vi "AlliGator Toggle Phasor Plot(s) Locking to Reference n.vi"(4 "Ref 1(F)/Ref 2(T)":bool, 6 "Phasor Frequency":dbl[unit], 7 "Phasor Graph Refnum":refnum<vi>, 8 "error in":errorcluster, 9 "State Indicators":refnum<vi>, 10 "Phasor Graph Ctrl Refnums":T1, 11 "[Phasor Plot(s) locked to Ref n] in":i32[](array[numeric])) -> (0 "error out":errorcluster, 3 "[Phasor Plot(s) locked to Ref n] out":i32[](array[numeric]))   [LabVIEW 2021, in "AlliGator Phasor Graph.lvlib"]
doc: "Locks Phasor Plot(s) to a reference."
uses:
  AlliGator Phasor Graph.lvlib
  AlliGator Phasor Graph Ctrl Refnums.ctl
  Phasor/Phasor Calibration Type.ctl
  AlliGator State Indicator.ctl
  AlliGator Variables List.ctl
  AlliGator Globals, Variables & Constants.lvlib
  Graphs/XY Graph/XY Graph Add-Ons.lvlib
  Sound/Sound.lvlib
  Phasor/Phasor.lvlib
  AlliGator GUI.lvlib
panel:
  # "see the AlliGator License on the block diagram (Ctrl+E or Window:Show Block Diagram)"
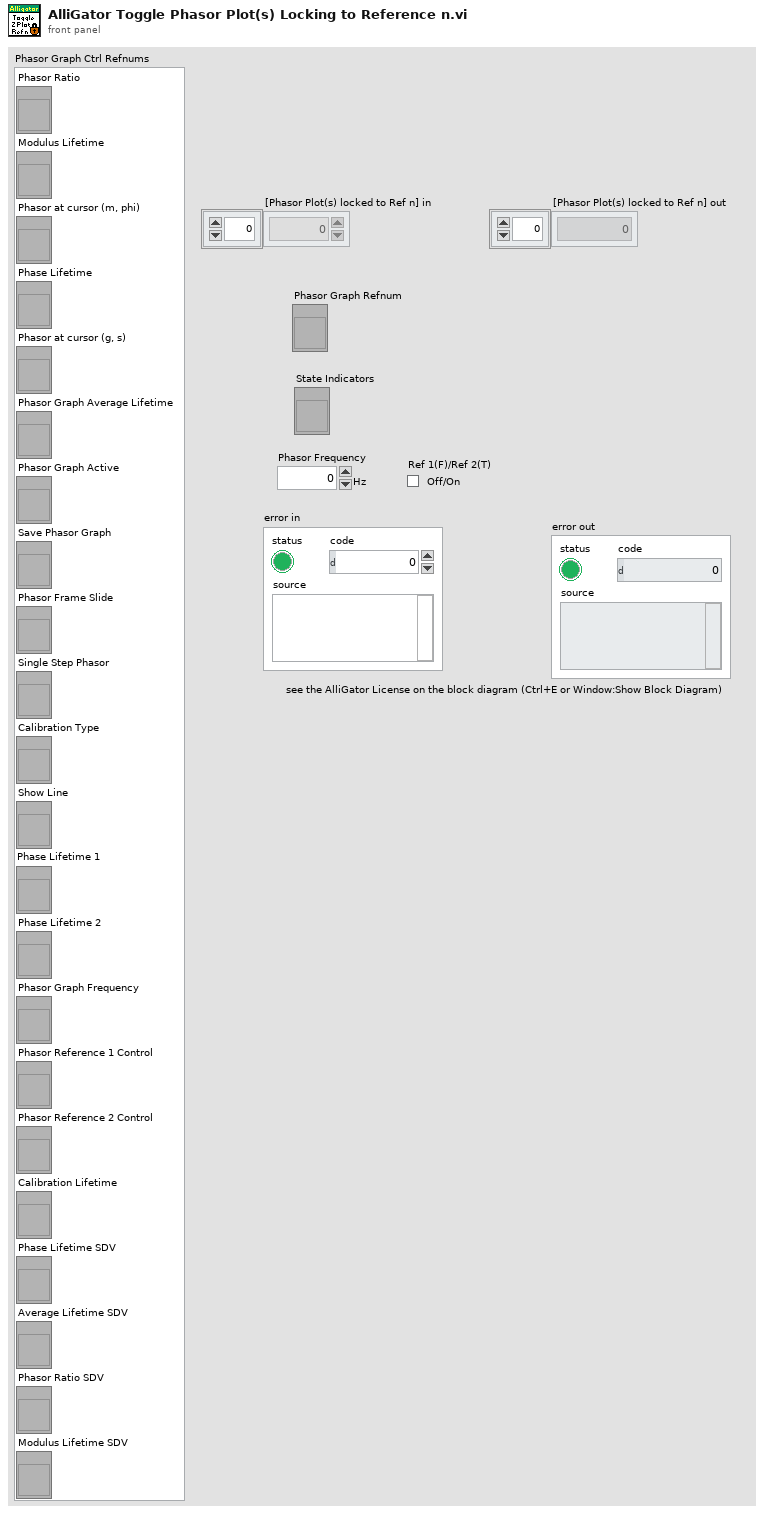
[diagram p1: front panel]
types:
  T1 = typedef "AlliGator GUI.lvlib/AlliGator Phasor Graph Ctrl Refnums.ctl" = cluster{"Phasor Ratio":refnum<vi>, "Modulus Lifetime":refnum<vi>, "Phasor at cursor (m, phi)":refnum<vi>, "Phase Lifetime":refnum<vi>, "Phasor at cursor (g, s)":refnum<vi>, "Phasor Graph Average Lifetime":refnum<vi>, "Phasor Graph Active":refnum<vi>, "Save Phasor Graph":refnum<vi>, "Phasor Frame Slide":refnum<vi>, "Single Step Phasor":refnum<vi>, "Calibration Type":refnum<vi>, "Show Line":refnum<vi>, "Phase Lifetime 1":refnum<vi>, "Phase Lifetime 2":refnum<vi>, "Phasor Graph Frequency":refnum<vi>, "Phasor Reference 1 Control":refnum<vi>, "Phasor Reference 2 Control":refnum<vi>, "Calibration Lifetime":refnum<vi>, "Phase Lifetime SDV":refnum<vi>, "Average Lifetime SDV":refnum<vi>, "Phasor Ratio SDV":refnum<vi>, "Modulus Lifetime SDV":refnum<vi>}
  T2 = typedef "AlliGator Globals, Variables & Constants.lvlib/AlliGator Variables List.ctl" = enum16{"---- GUI ----", "Initialization Status", "State Indicators Refnum", "Original AlliGator Menu Items", "Current Action Loop State", "Script in progress", "Playback", "Loop Playback", "Search ROI Used", "Search ROI", "Decay Graph Max Legend Size", "Intensity Graph Max Legend Size", "Decay Statistics Graph Max Legend Size", "Phasor Graph Max Legend Size", "Phasor Ratio Graph Max Legend Size", "Lifetime Graph Max Legend Size", "---- Files ----", "Export Dataset Frames as Individual Files", "Show Batch Export Help Balloons", "Frames in Dataset", "ptu File Frame Start Indices", "Current Frame in Dataset", "Current Frame Timestamp", "------ Python Plugins ------", "Python Plugins Information", "Python Session", "Valid Python Session?", "---- Source Image ----", "Dataset Loaded", "Dataset Metadata", "Dataset Channel", "Dataset Data Description", "Background Dataset Metadata", "Background Dataset Channel", "Background Dataset Data Description", "Background File Subtraction", "Background File Path", "Background File Pile-up Correction", "Background File Pixel Well Capacity", "Background File Scaling Factor", "Source Image ROIs", "Current Source Image ROI", "Source Image ROI Event Refnum", "X_Source Image Display Range", "X_Source Image Palette Information", "Source Image Palette List", "Source Image Scale", "Current Dataset Load Settings", "Source Image:ROI Overlay Color", "---- Image Profile Window ----", "Image Profile:Overlay ROI in Source Image", "Image Profile Window Event Refnum", "Image Profile:IntensityType", "Image Profile:Intensity Average Type", "Image Profile:Intensity-weighted SDV", "Image Profile:Box Profile Type", "Image Profile Window Open", "Image Profile:Plotted Fit Parameter", "X_Type of Displayed Image", "X_Time Gate Slider", "Dataset Path", "Source Image Overlay to Erase", "Is Displayed Image Accumulated", "White Light Image Modified", "Mask Image Modified", "Macrotime Gate Separation", "------ Phasor Graph -------", "Phasor Graph:Show Line", "---- Phasor Plot ---", "Phasor Plot Parameters Changed", "FLI Dataset Modified since last Phasor Plot Calculation", "Phasor Harmonics Data", "Selected Phasor Harmonics", "Phasor Harmonic Manager Event Refnum", "Phasor Plot ROIs", "Current Phasor Plot ROI", "Phasor Plot ROI Event Refnum", "Phasor Plot Image Reference Points", "Phasor Plot Computed", "Phasor Plot Palette Information", "Phasor Plot Palette List", "Phasor Ratio Palette Information", "Phasor Ratio Palette List", "Phasor Image Scale", "Phasor Plot Image Overlay to Erase", "Phasor Plot Image Elements to Update", "Current Phasor Plot Calculation Parameters", "Current Phasor Calibration Options", "Reset Cumulated Phasor Plot", "Phasor Ratio Reference 1", "Phasor Ratio Lifetime Reference 1", "Phasor Ratio Reference 1 Frequency", "Phasor Ratio Reference 2", "Phasor Ratio Lifetime Reference 2", "Phasor Ratio Reference 2 Frequency", "---- Decay Analysis ----", "Number of Selected Decays to Fit", "LS Fit Results", "LAR Fit Results", "BS Fit Results", "Last Decay Max - Min", "Best Fit Parameters", "Best Fit Parameter Names", "Actual Size X", "Actual Size Y", "Binning X", "Binning Y", "Actual # Gates", "Dataset Number", "Gates to...", "Gates Skipped", "Gates to keep", "Gate Step", "Gate Separation", "Reversed Gates", "Pile-up Correction", "Pixel Well Capacity", "Background Subtracted", "Background Subtraction Method", "Background Definition Range", "Background File (deprecated)", "Number of Dataset Accumulated", "Array of Accumulated Dataset Paths", "Do Averaged Datasets", "Destination File Path", "Process Plot Target", "Use 1/D as Phasor Frequency", "---- Decay Fit Parameter Map -----", "Decay Fit Parameter Map Palette Information", "Decay Fit Parameter Map Palette List", "Local Decay Graph Window Event Refnum", "------- Local Decay Window ---------", "Use normalized IRF for convolution", "----- Miscellaneous ----", "Skippable Dialog Windows Status"}
  T3 = typedef "AlliGator State Indicator.ctl" = cluster{"Phasor Calibration Defined":bool, "Phasor Calibration Series Defined":bool, "Phasor Calibration Map Defined":bool, "Phasor Ratio Reference 1 Defined":bool, "Phasor Ratio Reference 2 Defined":bool, "Phasor Ratio Lifetime Reference 1 Defined ":bool, "Phasor Ratio Lifetime Reference 2 Defined":bool, "Phasor Calibration Used":bool, "Phasor Calibration Series Used":bool, "Phasor Calibration Map Used":bool, "Dataset Update Needed":bool, "Phasor Plot Update Needed":bool, "Reference/IRF Defined":bool, "Individual IRFs Defined":bool}
  T4 = typedef "Phasor.lvlib/Phasor (m, phi).ctl" = cluster{"m":dbl, "phi":dbl}
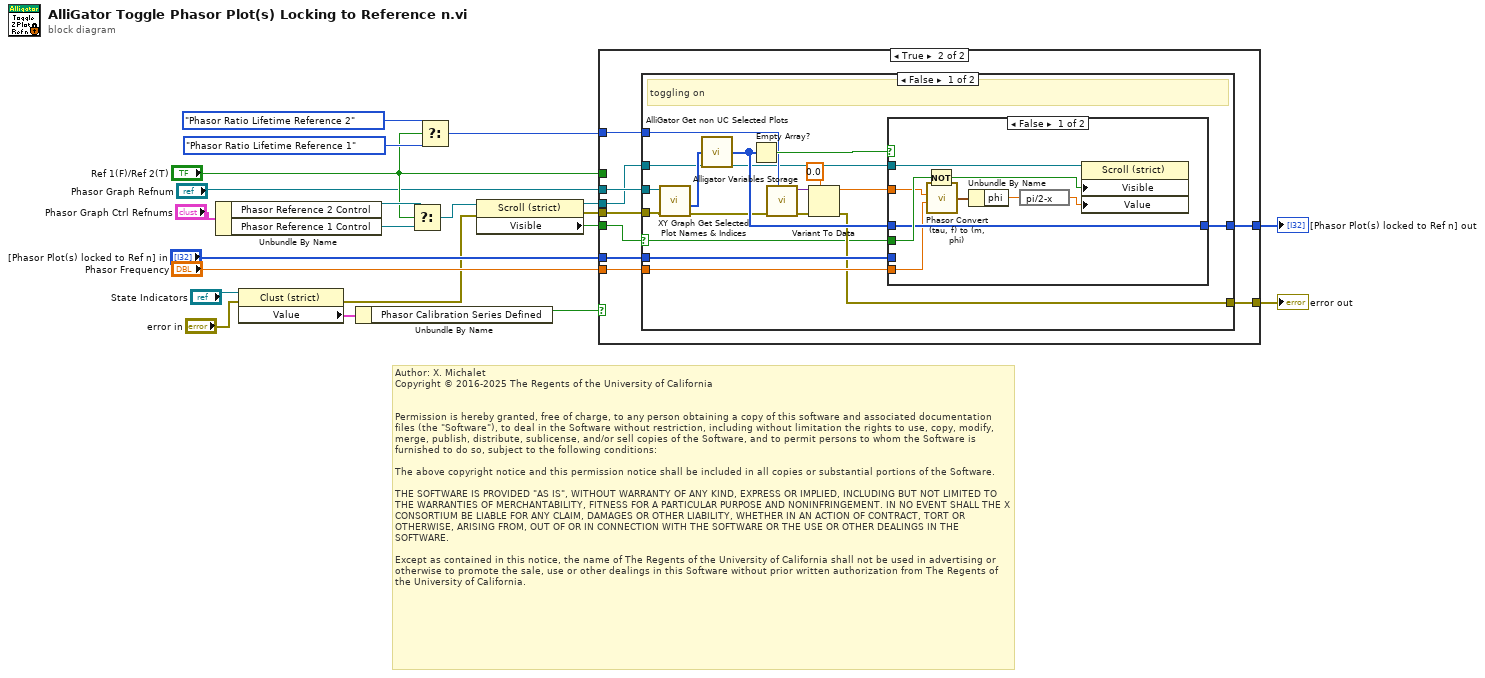
[diagram p0: block diagram]
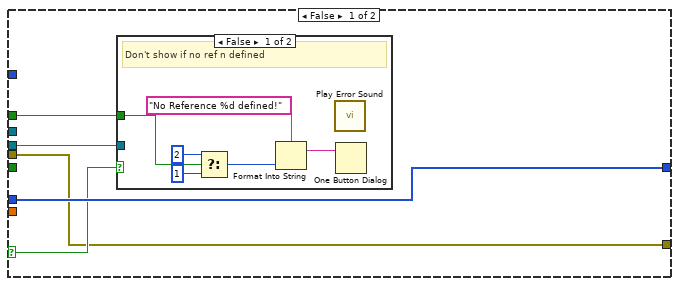
[diagram p2: hidden frame]
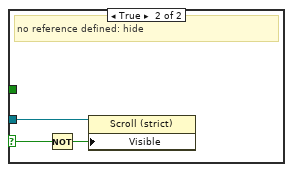
[diagram p3: hidden frame]
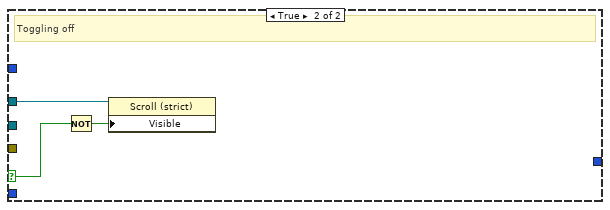
[diagram p5: hidden frame]
diagram:
  # "Author: X. Michalet\nCopyright © 2016-2025 The Regents of the University of California\n \n\nPermission is hereby granted, free of charge, to any person obtaining a copy of this software and associated documentation files (the \"Software\"), to deal in the Software without restriction, including without limitation the rights to use, copy, modify, merge, publish, distribute, sublicense, and/or sell copies of the Software, and to permit persons to whom the Software is furnished to do so, subject to the following conditions:\n\nThe above copyright notice and this permission notice shall be included in all copies or substantial portions of the Software.\n\nTHE SOFTWARE IS PROVIDED \"AS IS\", WITHOUT WARRANTY OF ANY KIND, EXPRESS OR IMPLIED, INCLUDING BUT NOT LIMITED TO THE WARRANTIES OF MERCHANTABILITY, FITNESS FOR A PARTICULAR PURPOSE AND NONINFRINGEMENT. IN NO EVENT SHALL THE X CONSORTIUM BE LIABLE FOR ANY CLAIM, DAMAGES OR OTHER LIABILITY, WHETHER IN AN ACTION OF CONTRACT, TORT OR OTHERWISE, ARISING FROM, OUT OF OR IN CONNECTION WITH THE SOFTWARE OR THE USE OR OTHER DEALINGS IN THE SOFTWARE.\n\nExcept as contained in this notice, the name of The Regents of the University of California shall not be used in advertising or otherwise to promote the sale, use or other dealings in this Software without prior written authorization from The Regents of the University of California."
  n1 = Unbundle By Name("Phasor Graph Ctrl Refnums") -> ("Phasor Reference 2 Control"=w7:refnum<vi>, "Phasor Reference 1 Control"=w8:refnum<vi>)
  n2 = property on="Property Node" class="Clust (strict)"(reference="State Indicators", error in="error in") -> (error out=w10:errorcluster, "Value"=w15:T3)  [unwired: 1 out]
  n3 = Unbundle By Name(w15) -> ("Phasor Calibration Series Defined"=w14:bool)
  n4 = Select(t=w7, s="Ref 1(F)/Ref 2(T)", f=w8) -> (s? t:f=w6:refnum<vi>)
  n5 = Select(t=AlliGator_Variables_List."Phasor Ratio Lifetime Reference 2" ("Alligator Variable"), s="Ref 1(F)/Ref 2(T)", f=AlliGator_Variables_List."Phasor Ratio Lifetime Reference 1" ("Alligator Variable")) -> (s? t:f=w3:T2)
  n6 = property on="Property Node" class="Scroll (strict)"(reference=w6, error in=w10) -> (reference out=w12:refnum<vi>, error out=w9:errorcluster, "Visible"=w13:bool)
  n7 = case shown="True" w14 {
    selector: w14 -> [w25 _]
    tunnel: "[Phasor Plot(s) locked to Ref n] in" -> [w26 w44]
    tunnel: [w26 w43] -> w19
    tunnel: "Phasor Frequency" -> [_ w42]
    tunnel: "Phasor Graph Refnum" -> [_ w41]
    tunnel: [w23 w40] -> w21
    tunnel: w13 -> [_ w39]
    tunnel: w12 -> [w24 w38]
    tunnel: w9 -> [w23 w37]
    tunnel: w3 -> [_ w36]
    tunnel: "Ref 1(F)/Ref 2(T)" -> [w22 _]
    frame False {
      n8 = case shown="False" w25 {
        selector: w25 -> [_ w35]
        tunnel: w24 -> [_ w33]
        tunnel: w22 -> [w30 _]
        frame False {
          # "Don't show if no ref n defined"
          n9 = Select(t=2, s=w30, f=1) -> (s? t:f=w27:i32)
          n10 = Format Into String(format string="No Reference %d defined!" ("message"), w27) -> (resulting string=w31:string)  [unwired: 2 in, 1 out]
          n11 = call "Play Error Sound.vi"() -> ()  [unwired: 27 in, 1 out]
          n12 = One Button Dialog(message=w31) -> ()  [unwired: 1 in, 1 out]
        }
        frame True {
          # "no reference defined: hide"
          n13 = Not(x=w35) -> (.not. x?=w34:bool)
          n14 = property on="Property Node" class="Scroll (strict)"(reference=w33, "Visible"=w34) -> ()  [unwired: 1 in, 2 out]
        }
      }
    }
    frame True {
      n15 = case shown="False" w39 {
        selector: w39 -> [w46 w72]
        tunnel: w44 -> [w60 _]
        tunnel: [w61 _] -> w43
        tunnel: w41 -> [w59 _]
        tunnel: w42 -> [w55 _]
        tunnel: w36 -> [w54 _]
        tunnel: [w49 _] -> w40
        tunnel: w38 -> [w47 w73]
        tunnel: w37 -> [w45 _]
        frame False {
          # "toggling on"
          n16 = call "XY Graph Get Selected Plot Names & Indices.vi"("error in (no error)"=w45, "XYGraph in"=w59) -> ("error out"=w48:errorcluster, "Selected Plots"=w58:i32[])  [unwired: 5 in, 3 out]
          n17 = call "AlliGator Get non UC Selected Plots.vi"("Selected Plots"=w58) -> ("Selected Plots - UC"=w56:i32[])  [unwired: 8 in]
          n18 = Empty Array?(array=w56) -> (empty?=w57:bool)
          n19 = call "Alligator Variables Storage.vi"("AlliGator Variable"=w54, "Error In"=w48) -> ("Error Out"=w52:errorcluster, "Data out"=w53:variant)  [unwired: 7 in, 1 out]
          n20 = Variant To Data(error in=w52, type=dbl[unit] 0.0 ("Lifetime"), Variant=w53) -> (data=w50:dbl[unit], error out=w49:errorcluster)
          n21 = case shown="False" w57 {
            tunnel: w46 -> [w69 _]
            tunnel: [w66 w71] -> w61
            tunnel: w60 -> [_ w71]
            tunnel: w56 -> [w66 _]
            tunnel: w55 -> [w65 _]
            tunnel: w50 -> [w64 _]
            tunnel: w47 -> [w62 _]
            frame False {
              n22 = Not(x=w69) -> (.not. x?=w70:bool)
              n23 = call "Phasor Convert (tau, f) to (m, phi).vi"("Lifetime"=w64, "Phasor Frequency"=w65) -> ("Phasor (m, phi)"=w68:T4)  [unwired: 5 in]
              n24 = Unbundle By Name(w68) -> ("phi"=w63:dbl)
              n25 = expression code="pi/2-x"(w63) -> (w67:dbl)
              n26 = property on="Property Node" class="Scroll (strict)"(reference=w62, "Visible"=w70, "Value"=w67) -> ()  [unwired: 1 in, 2 out]
            }
            frame True {
              # "UC: ignore"
            }
          }
        }
        frame True {
          # "Toggling off"
          n27 = Not(x=w72) -> (.not. x?=w74:bool)
          n28 = property on="Property Node" class="Scroll (strict)"(reference=w73, "Visible"=w74) -> ()  [unwired: 1 in, 2 out]
        }
      }
    }
  }
  "error out" <- w21
  "[Phasor Plot(s) locked to Ref n] out" <- w19
